vi "Cal RHS (Numeric).vi"(8 "error in (no error)":errorcluster, 10 "RHS in":variant, 11 "Domain_Steady_2D_Rect in":refnum<class "NI_Domain_Steady_2D_Rect.lvclass">) -> (0 "error out":errorcluster, 2 "RHS out":variant, 3 "Domain_Steady_2D_Rect out":refnum<class "NI_Domain_Steady_2D_Rect.lvclass">)   [LabVIEW 2020, in "NI_PDE.lvlib" / "NI_Domain_Steady_2D_Rect.lvclass"]
uses:
  <vilib>/gmath/pde.llb/DomainClass/Domain_Steady_2D_Rect/NI_Domain_Steady_2D_Rect.lvclass
  <vilib>/gmath/pde.llb/DomainClass/Domain_Steady_2D_Rect/NI_Domain_Steady_2D_Rect.lvclass/NI_Domain_Steady_2D_Rect.ctl
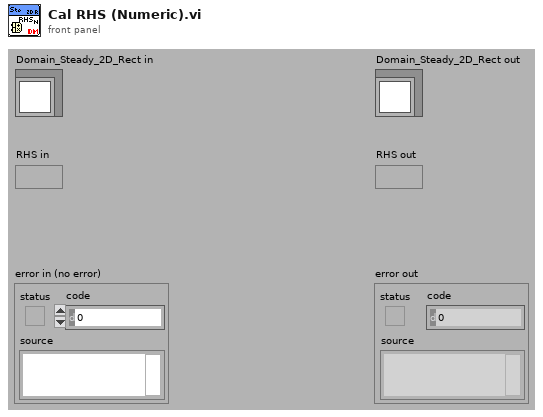
[diagram p1: front panel]
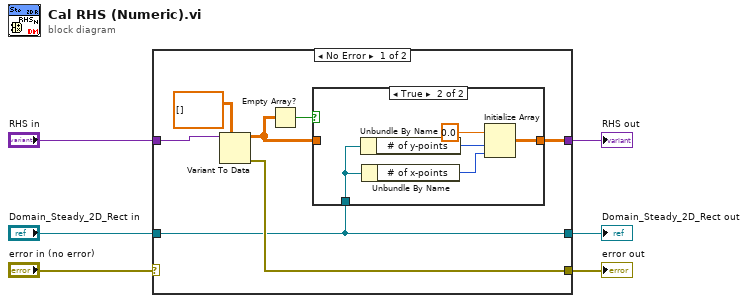
[diagram p0: block diagram]
diagram:
  n1 = case shown="No Error" "error in (no error)" {
    selector: "error in (no error)" -> [_ w22]
    tunnel: "Domain_Steady_2D_Rect in" -> [w7 w21]
    tunnel: [w7 w21] -> w6
    tunnel: [w8 w22] -> w5
    tunnel: [w13 w20] -> w2
    tunnel: "RHS in" -> [w12 w20]
    frame No Error {
      n2 = Variant To Data(type=dbl[][] [] ("F"), Variant=w12) -> (data=w10:dbl[][], error out=w8:errorcluster)  [unwired: 1 in]
      n3 = Empty Array?(array=w10) -> (empty?=w9:bool)
      n4 = case shown="True" w9 {
        tunnel: w7 -> [_ w15]
        tunnel: [w14 w16] -> w13
        tunnel: w10 -> [w14 _]
        frame False {
        }
        frame True {
          n5 = Unbundle By Name(w15) -> ("# of y-points"=w19:i32)
          n6 = Unbundle By Name(w15) -> ("# of x-points"=w18:i32)
          n7 = Initialize Array(0.0 ("element"), w19, w18) -> (w16:dbl[][])
        }
      }
    }
    frame Error {
    }
  }
  "Domain_Steady_2D_Rect out" <- w6
  "error out" <- w5
  "RHS out" <- w2
